vi "SensorReadings.vi"() -> ()   [LabVIEW 2018]
panel:
  out "LimeLight Distance (in)":dbl
  out "LimeLight Valid":bool
  out "Tank Pressure (PSI)":dbl
  out "Control Loop Time (ms)":u32
  out "Critical Pressure":bool
  out "Lower Intake Current (A)":dbl
  out "Upper Intake Current (A)":dbl
  in  "Range Color Front-Left":u32(colorbox)
  out "Front-Left Prox Sensor (in)":dbl format="%#_4g"
  out "Lower Pressure Transducer (V)":dbl
  out "Upper Pressure Transducer (V)":dbl
  out "Elevator Encoder Malfunction":bool
  out "EncoderVel_Elevator":dbl
  out "Hatch Captured":bool
  out "EncoderPos_Elevator":dbl
  out "Cargo Captured":bool
  in  "Range Color Front-Right":u32(colorbox)
  in  "Range Color Left":u32(colorbox)
  in  "Range Color Right":u32(colorbox)
  in  "Range Color Rear":u32(colorbox)
  out "Rear Prox Sensor (in)":dbl format="%#_4g"
  out "Front-Right Prox Sensor (in)":dbl format="%#_4g"
  out "Left Prox Sensor (in)":dbl format="%#_4g"
  out "LimeLight tx":dbl
  out "LimeLight ty":dbl
  out "Right Prox Sensor (in)":dbl format="%#_4g"
  out "EncoderVel_RightDrive":dbl
  out "EncoderVel_LeftDrive":dbl
  out "EncoderPos_RightDrive":dbl
  out "EncoderPos_LeftDrive":dbl
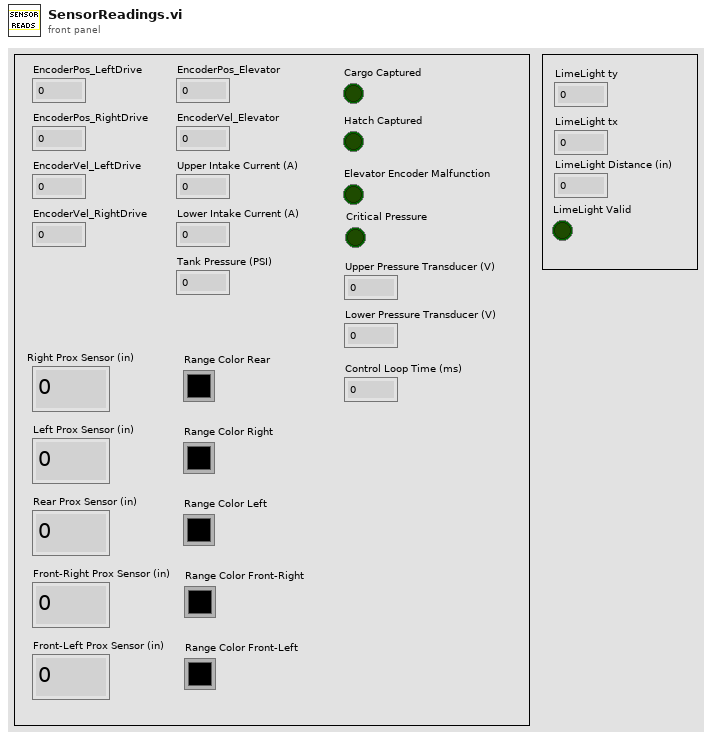
[diagram p1: front panel]
diagram:
